vi "DSF.Shared.Configuration.Transfer Group.Initialize.vi"(4 "Priority":u8, 6 "Cycle Timing Factors":T1={"Decimation"=1, "Offset"=0}, 7 "Custom Parameters":variant, 8 "error in (no error)":errorcluster, 9 "Transfer Configurations":refnum<class "DSF.Shared.Configuration.Transfer.lvclass">[](array[class]), 10 "Name":string, 11 "Transfer Group Configuration in":refnum<class "DSF.Shared.Configuration.Transfer Group.lvclass">) -> (0 "error out":errorcluster, 3 "Transfer Group Configuration out":refnum<class "DSF.Shared.Configuration.Transfer Group.lvclass">)   [LabVIEW 2016, in "DSF.Shared.lvlib" / "DSF.Shared.Configuration.Transfer Group.lvclass"]
uses:
  DSF.Shared.Configuration.Transfer Group.lvclass
  Typedefs/DSF.Shared.Typedefs.Cycle Timing Factors.ctl
  Transfer/DSF.Shared.Configuration.Transfer.lvclass
  DSF.Shared.Configuration.Transfer Group.lvclass/DSF.Shared.Configuration.Transfer Group.ctl
  DSF.Shared.lvlib
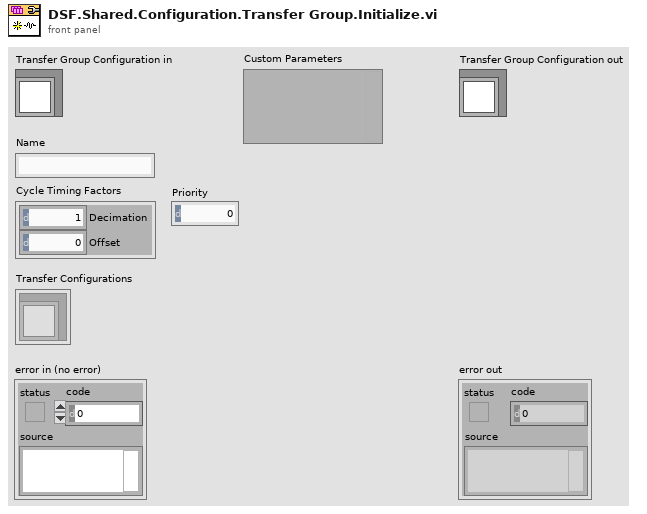
[diagram p1: front panel]
types:
  T1 = typedef "DSF.Shared.lvlib/DSF.Shared.Typedefs.Cycle Timing Factors.ctl" = cluster{"Decimation":u64, "Offset":u64}
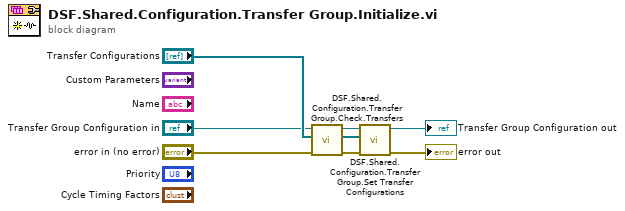
[diagram p0: block diagram]
diagram:
  n1 = call "DSF.Shared.Configuration.Transfer Group.Check.Transfers.vi"("error in (no error)"="error in (no error)", "Transfer Configurations in"="Transfer Configurations", "Transfer Group Configuration in"="Transfer Group Configuration in") -> ("error out"=w3:errorcluster, "Transfer Configurations out"=w4:refnum<class "DSF.Shared.Configuration.Transfer.lvclass">[], "Transfer Group Configuration out"=w5:refnum<class "DSF.Shared.Configuration.Transfer Group.lvclass">)  [unwired: 6 in]
  n2 = call "DSF.Shared.Configuration.Transfer Group.Set Transfer Configurations.vi"("error in (no error)"=w3, "Transfer Configurations"=w4, "Transfer Group Configuration in"=w5) -> ("error out"=→"error out":errorcluster, "Transfer Group Configuration out"=→"Transfer Group Configuration out":refnum<class "DSF.Shared.Configuration.Transfer Group.lvclass">)  [unwired: 7 in]
